vi "FormatDictionarySet.vi"(1 "value":string, 2 "key":string, 3 "dictionary":string) -> (0 "python object":string)   [LabVIEW 2014, in "Raspberry Pi Compatible Compiler for LabVIEW.lvlib" / "Python Functions.lvlib"]
uses:
  Python Functions.lvlib
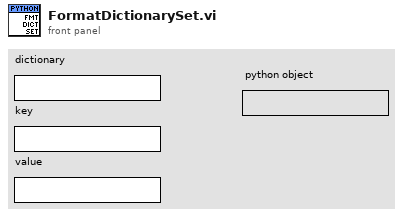
[diagram p1: front panel]
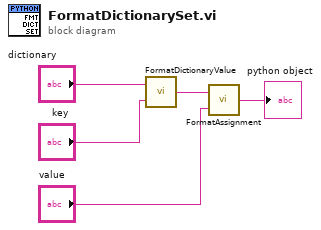
[diagram p0: block diagram]
diagram:
  n1 = call "FormatDictionaryValue.vi"("key"="key", "dictionary"="dictionary") -> ("python object"=w3:string)
  n2 = call "FormatAssignment.vi"("value"="value", "name"=w3) -> ("python assignment"=→"python object":string)
